vi "monitorRun.vi"(8 "error in (no error)":errorcluster) -> ()   [LabVIEW 2012]
uses:
  <vilib>/addons/database/Auxilliary.llb/DB Tools Cursor Type.ctl
  Global1.vi
  <vilib>/addons/database/Connection.llb/DB Tools Open Connec (Path).vi
  <vilib>/addons/database/Connection.llb/Conn Execute.vi
  <vilib>/addons/database/Recordset.llb/Rec Fetch Recordset Data (R).vi
  <vilib>/addons/database/Recordset.llb/Rec Destroy - Connection.vi
  <vilib>/addons/database/_DB Variant To Data/Database Variant To Data.xnode
  <vilib>/addons/database/NI_Database_API.lvlib
panel:
  out "error out":errorcluster
  out "M100 Monitor Board 2":string[][](table)
  in  "Table Control":string[][](table)
  out "error out 2":errorcluster
  in  "input cluster 2":T1
  in  "M100 Monitor Board":string[][](table)
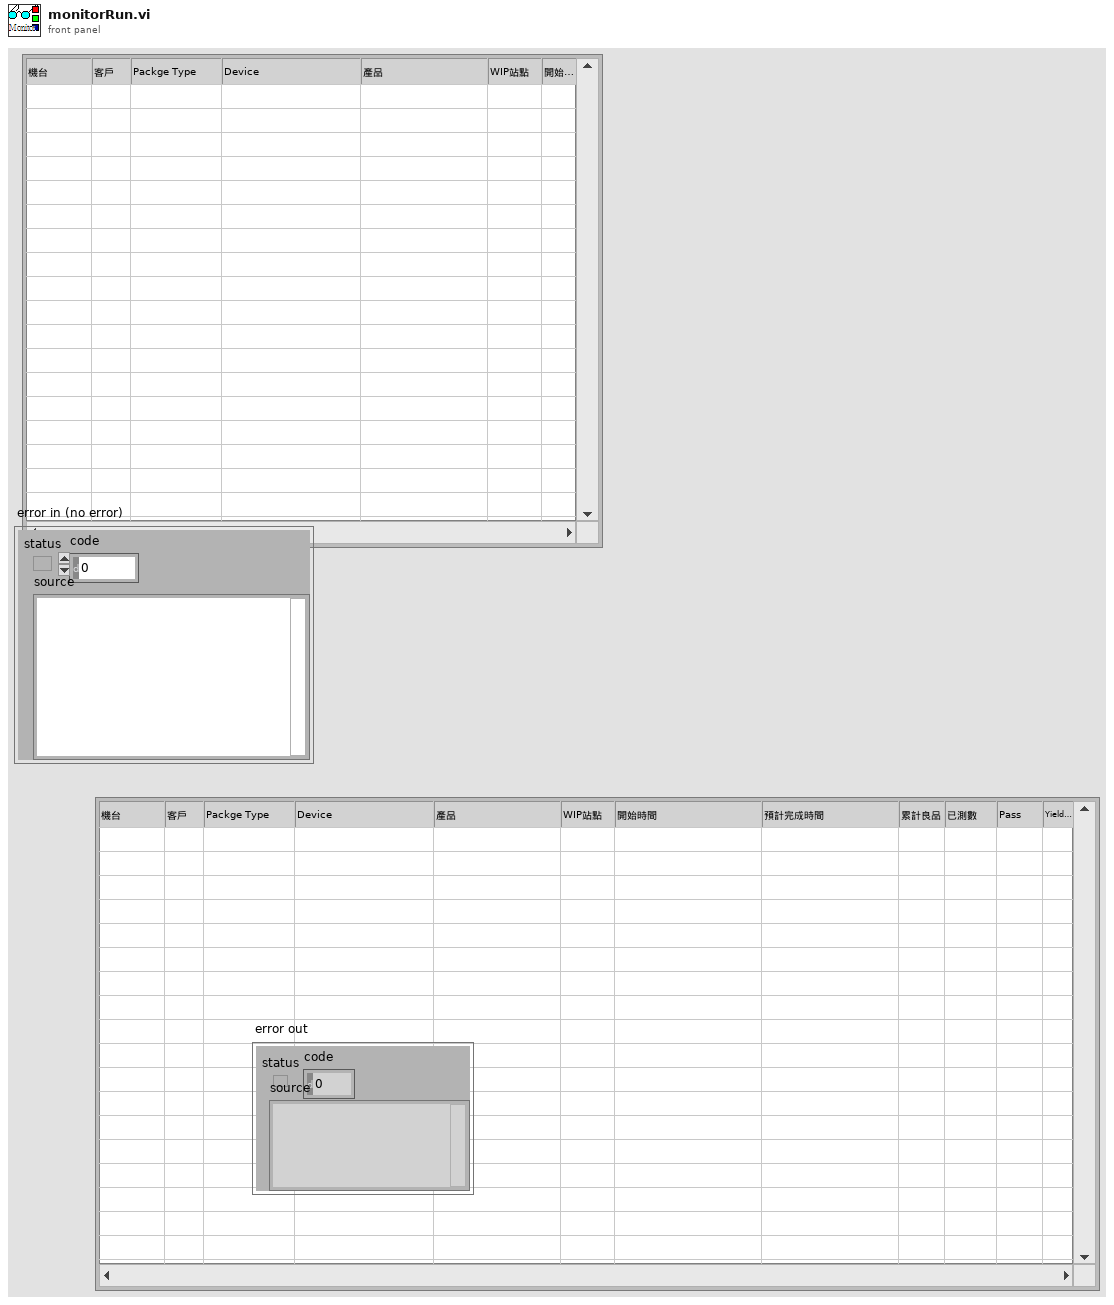
[diagram p1: front panel]
types:
  T1 = cluster{"Customer":string, "Package":string, "machine":string}
  T2 = typedef "NI_Database_API.lvlib/DB Tools Cursor Type.ctl" = enum16{"forward-only", "keyset", "dynamic", "static"}
  T3 = typedef "NI_Database_API.lvlib/Conn ObjectReference.ctl" = refnum<k1>
  T4 = typedef "LVDateTimeRec.ctl" = cluster{"fractional second":dbl, "second":i32, "minute":i32, "hour":i32, "day of month":i32, "month":i32, "year":i32, "day of week":i32, "day of year":i32, "DST":i32}
  T5 = typedef "LVRowAndColumnTypeDef.ctl" = cluster{"Row":i32, "Column":i32}
  T6 = typedef "NI_Database_API.lvlib/Rec ObjectReference.ctl" = refnum<k1>
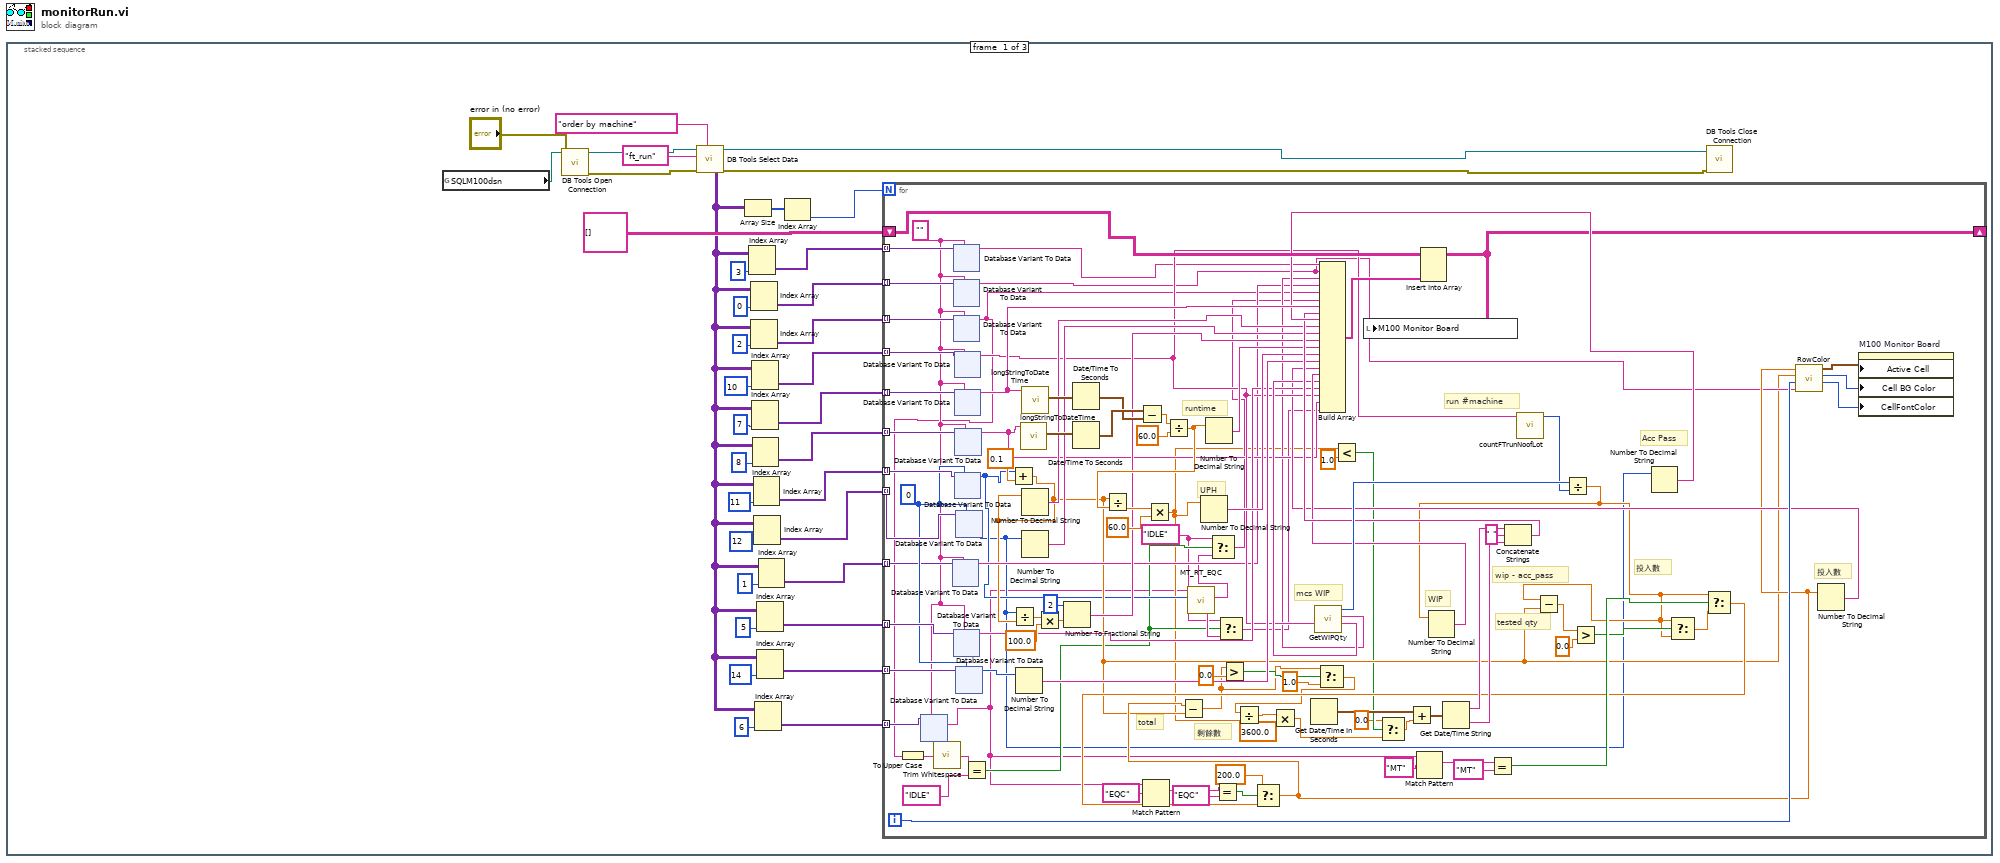
[diagram p0: block diagram]
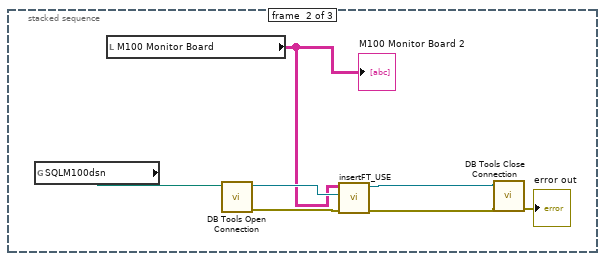
[diagram p2: hidden frame]
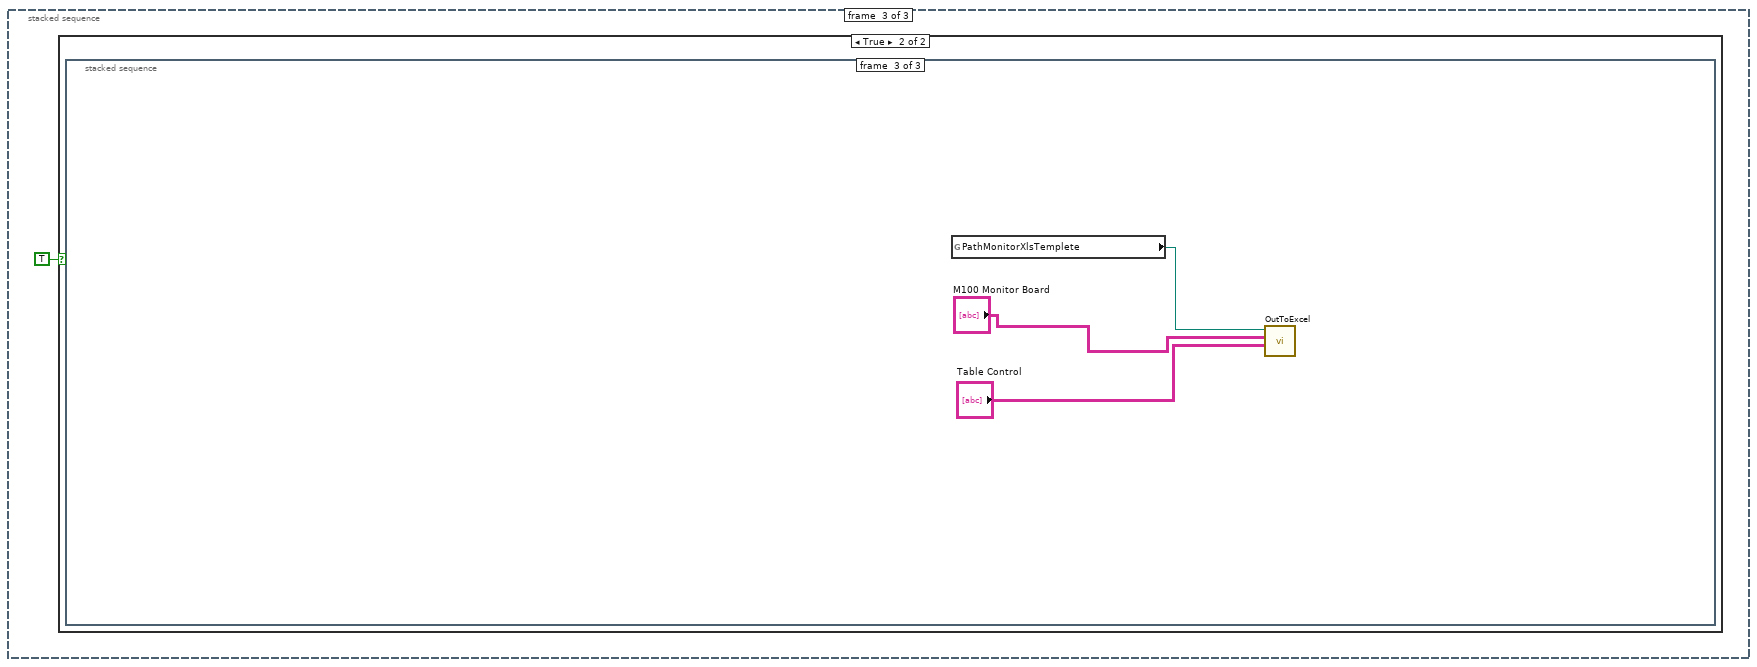
[diagram p3: hidden frame]
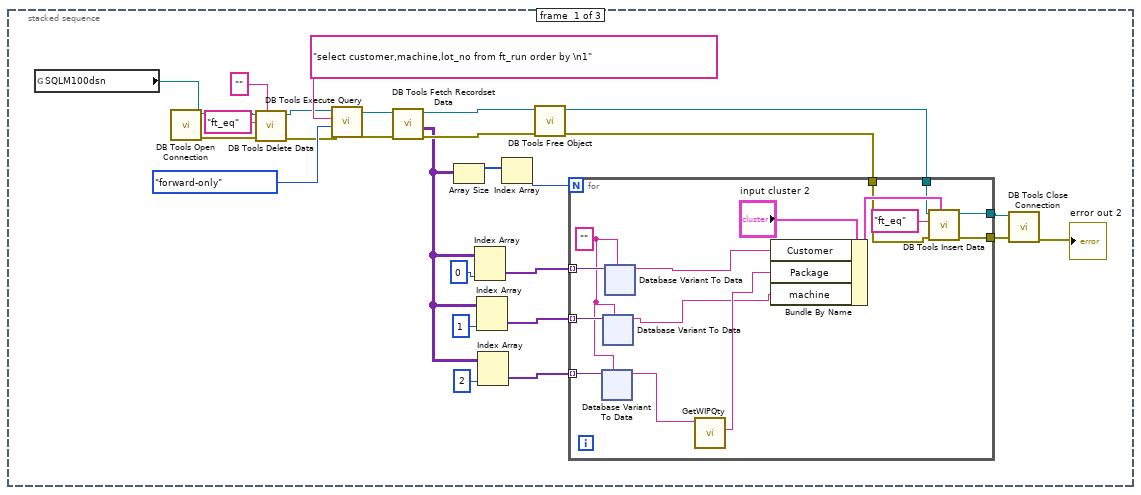
[diagram p5: hidden frame]
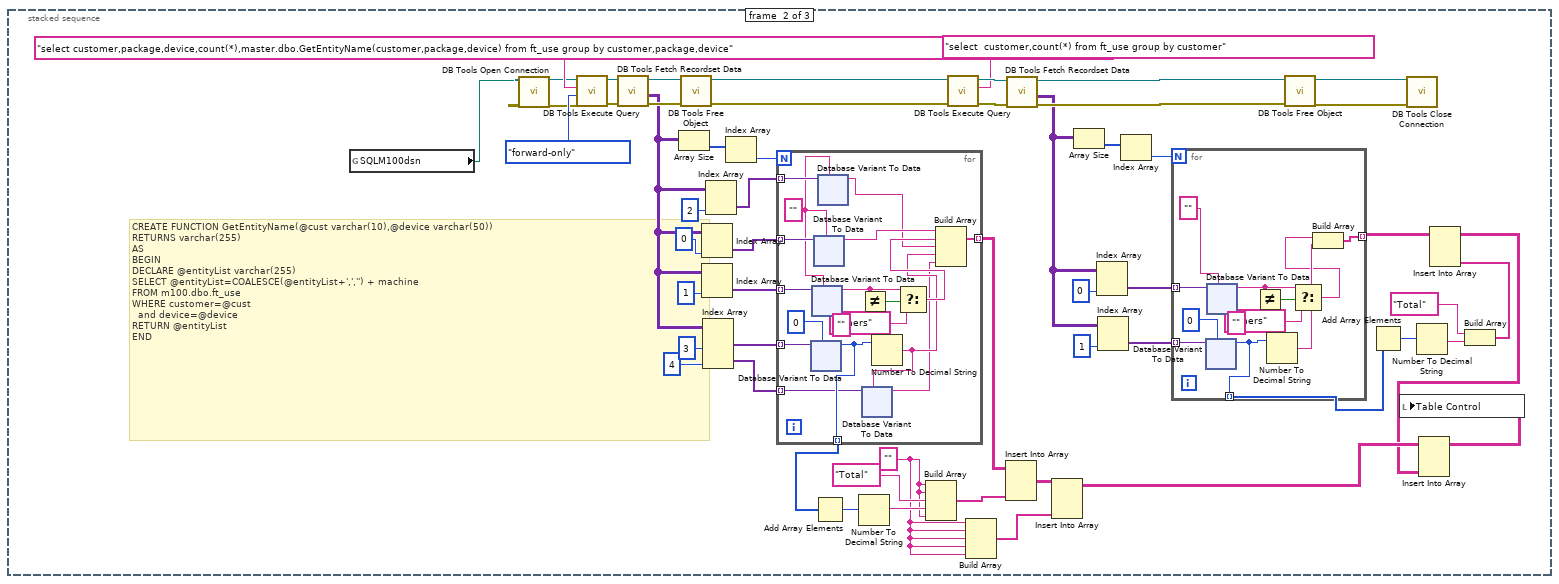
[diagram p6: hidden frame]
diagram:
  n1 = stacked-sequence {
    frame #0 {
      n2 = global read "Global1.vi" "SQLM100dsn"() -> (w4:path)
      n3 = call-poly <vilib>:"DB Tools Open Connection.vi"("error in (no error)"="error in (no error)", "connection information"=w4) -> ("error out"=w35:errorcluster, "connection reference"=w36:T3)  [unwired: 6 in]
      n4 = call <vilib>:"DB Tools Select Data.vi"("condition"="order by machine", "error in (no error)"=w35, "table"="ft_run", "connection reference"=w36) -> ("error out"=w6:errorcluster, "data"=w3:variant[][], "connection reference out"=w7:T3)  [unwired: 2 in]
      n5 = Array Size(array=w3) -> (size(s)=w33:i32[])
      n6 = Index Array(array=w3, index (col)=3) -> (element=w22:variant[])  [unwired: 1 in]
      n7 = Index Array(array=w3, index (col)=0) -> (element=w29:variant[])  [unwired: 1 in]
      n8 = Index Array(array=w3, index (col)=2) -> (element=w21:variant[])  [unwired: 1 in]
      n9 = Index Array(array=w3, index (col)=10) -> (element=w20:variant[])  [unwired: 1 in]
      n10 = Index Array(array=w3, index (col)=7) -> (element=w19:variant[])  [unwired: 1 in]
      n11 = Index Array(array=w3, index (col)=8) -> (element=w15:variant[])  [unwired: 1 in]
      n12 = Index Array(array=w3, index (col)=11) -> (element=w18:variant[])  [unwired: 1 in]
      n13 = Index Array(array=w3, index (col)=12) -> (element=w17:variant[])  [unwired: 1 in]
      n14 = Index Array(array=w3, index (col)=6 ("disabled index (col)")) -> (element=w1:variant[])  [unwired: 1 in]
      n15 = Index Array(array=w3, index (col)=5) -> (element=w13:variant[])  [unwired: 1 in]
      n16 = Index Array(array=w3, index (col)=14 ("disabled index (col)")) -> (element=w11:variant[])  [unwired: 1 in]
      n17 = Index Array(array=w3, index (col)=1 ("disabled index (col)")) -> (element=w8:variant[])  [unwired: 1 in]
      n18 = Index Array(array=w33) -> (element=w32:i32)  [unwired: 1 in]
      n19 = for {
        N: w32 -> [_]
        tunnel: w29 -> [w137] mode=indexing
        tunnel: w17 -> [w141] mode=indexing
        shift-right: [w72] -> _
        shift-left: string[][] [] -> [w140]
        tunnel: w22 -> [w138] mode=indexing
        tunnel: w21 -> [w136] mode=indexing
        tunnel: w20 -> [w135] mode=indexing
        tunnel: w19 -> [w134] mode=indexing
        tunnel: w18 -> [w133] mode=indexing
        tunnel: w15 -> [w129] mode=indexing
        tunnel: w13 -> [w119] mode=indexing
        tunnel: w11 -> [w118] mode=indexing
        tunnel: w8 -> [w77] mode=indexing
        tunnel: w1 -> [w58] mode=indexing
        i -> [w105]
        w50 = "IDLE" ("t")
        w117 = 0
        w57 = ""
        # "tested qty"
        # "wip - acc_pass"
        # "投入數"
        # "剩餘數"
        # "WIP"
        # "mcs WIP"
        # "run #machine"
        # "Acc Pass"
        # "total"
        # "UPH"
        # "runtime"
        # "投入數"
        n20 = xnode "Database Variant To Data"("database variant"=w58, "type"=w57) -> ("data"=w40:string)  [unwired: 1 in, 1 out]
        n21 = xnode "Database Variant To Data"("database variant"=w77, "type"=w57) -> ("data"=w73:string)  [unwired: 1 in, 1 out]
        n22 = xnode "Database Variant To Data"("database variant"=w138, "type"=w57) -> ("data"=w76:string)  [unwired: 1 in, 1 out]
        n23 = xnode "Database Variant To Data"("database variant"=w137, "type"=w57) -> ("data"=w75:string)  [unwired: 1 in, 1 out]
        n24 = xnode "Database Variant To Data"("database variant"=w136, "type"=w57) -> ("data"=w39:string)  [unwired: 1 in, 1 out]
        n25 = To Upper Case(1:w39) -> (0:w38:string)
        n26 = call <vilib>:"Trim Whitespace.vi"("string"=w38) -> ("trimmed string"=w37:string)  [unwired: 1 in]
        n27 = xnode "Database Variant To Data"("database variant"=w119, "type"=w57) -> ("data"=w91:string)  [unwired: 1 in, 1 out]
        n28 = xnode "Database Variant To Data"("database variant"=w135, "type"=w57) -> ("data"=w90:string)  [unwired: 1 in, 1 out]
        n29 = xnode "Database Variant To Data"("database variant"=w134, "type"=w57) -> ("data"=w102:string)  [unwired: 1 in, 1 out]
        n30 = xnode "Database Variant To Data"("database variant"=w133, "type"=w117) -> ("data"=w59:i32)  [unwired: 1 in, 1 out]
        n31 = xnode "Database Variant To Data"("database variant"=w129, "type"=w57) -> ("data"=w88:string)  [unwired: 1 in, 1 out]
        n32 = xnode "Database Variant To Data"("database variant"=w141, "type"=w117) -> ("data"=w45:i32)  [unwired: 1 in, 1 out]
        n33 = xnode "Database Variant To Data"("database variant"=w118, "type"=w117) -> ("data"=w116:i32)  [unwired: 1 in, 1 out]
        n34 = Equal?(x=w37, y="IDLE") -> (x = y?=w51:bool)
        n35 = Add(x=w59, y=0.1) -> (x+y=w65:dbl)
        n36 = Divide(x=w45, y=w65) -> (x/y=w130:dbl)
        n37 = Number To Decimal String(number=w116) -> (decimal integer string=w94:string)  [unwired: 1 in]
        n38 = call "longStringToDateTime.vi"("input string"=w88) -> ("output cluster"=w128:T4)  [unwired: 10 in]
        n39 = call "longStringToDateTime.vi"("input string"=w102) -> ("output cluster"=w127:T4)  [unwired: 10 in]
        n40 = Number To Decimal String(number=w65) -> (decimal integer string=w99:string)  [unwired: 1 in]
        n41 = Number To Decimal String(number=w45) -> (decimal integer string=w98:string)  [unwired: 1 in]
        n42 = Multiply(x=w130, y=100.0) -> (x*y=w131:dbl)
        n43 = Number To Fractional String(number=w131, precision (6)=i16 2) -> (F-format string=w97:string)  [unwired: 2 in]
        n44 = Date/Time To Seconds(2:w127) -> (0:w125:timestamp)  [unwired: 1 in]
        n45 = Date/Time To Seconds(2:w128) -> (0:w126:timestamp)  [unwired: 1 in]
        n46 = Subtract(x=w126, y=w125) -> (x-y=w124:dbl)
        n47 = Match Pattern(string=w40, regular expression="EQC") -> (match substring=w86:string)  [unwired: 1 in, 3 out]
        n48 = Divide(x=w124, y=60.0) -> (x/y=w122:dbl)
        n49 = Divide(x=w65, y=w122) -> (x/y=w121:dbl)
        n50 = Multiply(x=w121, y=60.0) -> (x*y=w48:dbl)
        n51 = call "MT_RT_EQC.vi"("Qty"=w59, "input string"=w40) -> ("Station"=w54:string, "STN"=w52:string)  [unwired: 5 in, 3 out]
        n52 = Number To Decimal String(number=w48) -> (decimal integer string=w95:string)  [unwired: 1 in]
        n53 = Number To Decimal String(number=w122) -> (decimal integer string=w96:string)  [unwired: 1 in]
        n54 = Select(t=w50, s=w51, f=w54) -> (s? t:f=w55:string)
        n55 = Equal?(x=w86, y="EQC") -> (x = y?=w84:bool)
        n56 = Select(t=w50, s=w51, f=w52) -> (s? t:f=w53:string)
        n57 = Get Date/Time In Seconds() -> (seconds since 1Jan1904=w113:timestamp)
        n58 = call "GetWIPQty.vi"("Lotno"=w90) -> ("lotno"=w92:string, "Package"=w74:string, "data"=w104:i32)  [unwired: 2 in, 6 out]
        n59 = Less?(x=w48, y=1.0) -> (x < y?=w44:bool)
        n60 = Match Pattern(string=w40, regular expression="MT") -> (match substring=w82:string)  [unwired: 1 in, 3 out]
        n61 = Equal?(x=w82, y="MT") -> (x = y?=w80:bool)
        n62 = call "countFTrunNoofLot.vi"("Lotno"=w90) -> ("data"=w103:i32)  [unwired: 10 in]
        n63 = Divide(x=w104, y=w103) -> (x/y=w49:dbl)
        n64 = Number To Decimal String(number=w49) -> (decimal integer string=w93:string)  [unwired: 1 in]
        n65 = Subtract(x=w49, y=w65) -> (x-y=w68:dbl)
        n66 = Greater?(x=w68, y=0.0) -> (0:w70:bool)
        n67 = Number To Decimal String(number=w45) -> (decimal integer string=w101:string)  [unwired: 1 in]
        n68 = Select(t=w49, s=w70, f=w49) -> (s? t:f=w69:dbl)
        n69 = Select(t=w49, s=w80, f=w69) -> (s? t:f=w79:dbl)
        n70 = Select(t=200.0, s=w84, f=w79) -> (s? t:f=w78:dbl)
        n71 = Subtract(x=w78, y=w65) -> (x-y=w62:dbl)
        n72 = Greater?(x=w62, y=0.0) -> (0:w63:bool)
        n73 = Select(t=w62, s=w63, f=1.0) -> (s? t:f=w60:dbl)
        n74 = Divide(x=w60, y=w48) -> (x/y=w115:dbl)
        n75 = Multiply(x=w115, y=3600.0) -> (x*y=w42:dbl)
        n76 = Select(t=0.0, s=w44, f=w42) -> (s? t:f=w41:dbl)
        n77 = Add(x=w113, y=w41) -> (x+y=w112:timestamp)
        n78 = Get Date/Time String(seconds (now)=w112) -> (date string=w111:string, time string=w110:string)  [unwired: 2 in]
        n79 = Concatenate Strings(w111, " " ("string"), w110) -> (w100:string)
        n80 = call "RowColor.vi"("Customer"=w75, "Row"=w105, "tested"=w65, "Input"=w78) -> ("FontColor"=w106:u32, "bgcolor"=w107:u32, "ActiveCell"=w108:T5)  [unwired: 5 in]
        n81 = Number To Decimal String(number=w78) -> (decimal integer string=w89:string)  [unwired: 1 in]
        n82 = Build Array(w76, w75, w74, w73, w39, w55, w102, w100, w101, w99, w98, w97, w96, w95, w94, w89, w93, w92, w91, w90, w88, w53) -> (w139:string[])
        n83 = Insert Into Array(array=w140, new element=w139) -> (w72:string[][])  [unwired: 2 in]
        n84 = local write "M100 Monitor Board"(w72) -> ()
        n85 = property on="M100 Monitor Board" class="Tbl (strict)"("Active Cell"=w108, "Cell BG Color"=w107, "CellFontColor"=w106) -> ()  [unwired: 2 in, 2 out]
      }
      n86 = call <vilib>:"DB Tools Close Connection.vi"("error in (no error)"=w6, "connection reference"=w7) -> ()  [unwired: 5 in, 1 out]
    }
    frame #1 {
      n87 = global read "Global1.vi" "SQLM100dsn"() -> (w529:path)
      n88 = local read "M100 Monitor Board"() -> (w528:string[][])
      "M100 Monitor Board 2" <- w528
      n89 = call-poly <vilib>:"DB Tools Open Connection.vi"("connection information"=w529) -> ("error out"=w531:errorcluster, "connection reference"=w532:T3)  [unwired: 7 in]
      n90 = call "insertFT_USE.vi"("M100 Monitor Board"=w528, "connection reference"=w532, "error in (no error)"=w531) -> ("connection reference out"=w530:T3, "error out"=w526:errorcluster)  [unwired: 6 in]
      n91 = call <vilib>:"DB Tools Close Connection.vi"("error in (no error)"=w526, "connection reference"=w530) -> ("error out"=→"error out":errorcluster)  [unwired: 5 in]
    }
    frame #2 {
      n92 = case shown="True" TRUE {
        frame False {
        }
        frame True {
          n93 = stacked-sequence {
            frame #0 {
              n94 = global read "Global1.vi" "SQLM100dsn"() -> (w534:path)
              n95 = call-poly <vilib>:"DB Tools Open Connection.vi"("connection information"=w534) -> ("error out"=w545:errorcluster, "connection reference"=w546:T3)  [unwired: 7 in]
              n96 = call <vilib>:"DB Tools Delete Data.vi"("condition"="", "error in (no error)"=w545, "table"="ft_eq", "connection reference"=w546) -> ("error out"=w543:errorcluster, "connection reference out"=w542:T3)  [unwired: 6 in]
              n97 = call-poly <vilib>:"DB Tools Execute Query.vi"("error in (no error)"=w543, "cursor type"=DB_Tools_Cursor_Type."forward-only", "SQL query"="select customer,machine,lot_no from ft_run order by \n1", "connection reference"=w542) -> ("error out"=w558:errorcluster, "recordset reference"=w560:T6)  [unwired: 4 in]
              n98 = call-poly <vilib>:"DB Tools Fetch Recordset Data.vi"("error in (no error)"=w558, "recordset reference"=w560) -> ("error out"=w557:errorcluster, "recordset data"=w552:variant[][], "recordset reference out"=w559:T6)  [unwired: 3 in]
              n99 = Array Size(array=w552) -> (size(s)=w551:i32[])
              n100 = Index Array(array=w552, index (col)=0 ("disabled index (col)")) -> (element=w549:variant[])  [unwired: 1 in]
              n101 = Index Array(array=w552, index (col)=1 ("disabled index (col)")) -> (element=w548:variant[])  [unwired: 1 in]
              n102 = Index Array(array=w552, index (col)=2) -> (element=w547:variant[])  [unwired: 1 in]
              n103 = Index Array(array=w551) -> (element=w550:i32)  [unwired: 1 in]
              n104 = call-poly <vilib>:"DB Tools Free Object.vi"("error in (no error)"=w557, "recordset reference"=w559) -> ("error out"=w538:errorcluster, "connection reference"=w539:T3)  [unwired: 8 in]
              n105 = for {
                N: w550 -> [_]
                tunnel: w549 -> [w575] mode=indexing
                tunnel: w548 -> [w574] mode=indexing
                tunnel: w547 -> [w573] mode=indexing
                tunnel: w539 -> [w564]
                tunnel: w538 -> [w563]
                tunnel: [w562] -> w537
                tunnel: [w561] -> w536
                w572 = ""
                n106 = xnode "Database Variant To Data"("database variant"=w573, "type"=w572) -> ("data"=w571:string)  [unwired: 1 in, 1 out]
                n107 = xnode "Database Variant To Data"("database variant"=w574, "type"=w572) -> ("data"=w566:string)  [unwired: 1 in, 1 out]
                n108 = xnode "Database Variant To Data"("database variant"=w575, "type"=w572) -> ("data"=w568:string)  [unwired: 1 in, 1 out]
                n109 = call "GetWIPQty.vi"("Lotno"=w571) -> ("Package"=w567:string)  [unwired: 2 in, 8 out]
                n110 = Bundle By Name(cluster="input cluster 2", "Customer"=w568, "Package"=w567, "machine"=w566) -> (w565:T1)
                n111 = call <vilib>:"DB Tools Insert Data.vi"("data"=w565, "error in (no error)"=w563, "table"="ft_eq", "connection reference"=w564) -> ("error out"=w561:errorcluster, "connection reference out"=w562:T3)  [unwired: 6 in]
              }
              n112 = call <vilib>:"DB Tools Close Connection.vi"("error in (no error)"=w536, "connection reference"=w537) -> ("error out"=→"error out 2":errorcluster)  [unwired: 5 in]
            }
            frame #1 {
              w672 = "" ("element")
              # "CREATE FUNCTION GetEntityName(@cust varchar(10),@device varchar(50))\nRETURNS varchar(255) \nAS\nBEGIN\nDECLARE @entityList varchar(255)\nSELECT @entityList=COALESCE(@entityList+',','') + machine\nFROM m100.dbo.ft_use\nWHERE customer=@cust\n  and device=@device\nRETURN @entityList\nEND"
              n113 = global read "Global1.vi" "SQLM100dsn"() -> (w675:path)
              n114 = call-poly <vilib>:"DB Tools Open Connection.vi"("connection information"=w675) -> ("error out"=w716:errorcluster, "connection reference"=w717:T3)  [unwired: 7 in]
              n115 = call-poly <vilib>:"DB Tools Execute Query.vi"("error in (no error)"=w716, "cursor type"=DB_Tools_Cursor_Type."forward-only", "SQL query"="select customer,package,device,count(*),master.dbo.GetEntityName(customer,package,device) from ft_use group by customer,package,device", "connection reference"=w717) -> ("error out"=w725:errorcluster, "recordset reference"=w727:T6)  [unwired: 4 in]
              n116 = call-poly <vilib>:"DB Tools Fetch Recordset Data.vi"("error in (no error)"=w725, "recordset reference"=w727) -> ("error out"=w724:errorcluster, "recordset data"=w678:variant[][], "recordset reference out"=w726:T6)  [unwired: 3 in]
              n117 = Array Size(array=w678) -> (size(s)=w719:i32[])
              n118 = call-poly <vilib>:"DB Tools Free Object.vi"("error in (no error)"=w724, "recordset reference"=w726) -> ("error out"=w685:errorcluster, "connection reference"=w686:T3)  [unwired: 8 in]
              n119 = Index Array(array=w678, index (col)=0 ("disabled index (col)")) -> (element=w714:variant[])  [unwired: 1 in]
              n120 = Index Array(array=w678, index (col)=1 ("disabled index (col)")) -> (element=w713:variant[])  [unwired: 1 in]
              n121 = Index Array(array=w678, index (col) #1=3 ("index (col)"), index (col) #2=4 ("index (col)")) -> (element #1=w712:variant[], element #2=w673:variant[])  [unwired: 2 in]
              n122 = Index Array(array=w678, index (col)=2 ("disabled index (col)")) -> (element=w676:variant[])  [unwired: 1 in]
              n123 = Index Array(array=w719) -> (element=w715:i32)  [unwired: 1 in]
              n124 = for {
                N: w715 -> [_]
                tunnel: w714 -> [w821] mode=indexing
                tunnel: w713 -> [w820] mode=indexing
                tunnel: w712 -> [w819] mode=indexing
                tunnel: [w816] -> w707 mode=indexing
                tunnel: [w810] -> w710 mode=indexing
                tunnel: w676 -> [w809] mode=indexing
                tunnel: w673 -> [w806] mode=indexing
                w808 = ""
                n125 = xnode "Database Variant To Data"("database variant"=w819, "type"=0) -> ("data"=w810:i32)  [unwired: 1 in, 1 out]
                n126 = xnode "Database Variant To Data"("database variant"=w820, "type"=w808) -> ("data"=w813:string)  [unwired: 1 in, 1 out]
                n127 = xnode "Database Variant To Data"("database variant"=w821, "type"=w808) -> ("data"=w817:string)  [unwired: 1 in, 1 out]
                n128 = xnode "Database Variant To Data"("database variant"=w809, "type"=w808) -> ("data"=w807:string)  [unwired: 1 in, 1 out]
                n129 = Not Equal?(x=w813, y="") -> (x != y?=w814:bool)
                n130 = Number To Decimal String(number=w810) -> (decimal integer string=w805:string)  [unwired: 1 in]
                n131 = xnode "Database Variant To Data"("database variant"=w806, "type"=w805) -> ("data"=w804:string)  [unwired: 1 in, 1 out]
                n132 = Select(t=w813, s=w814, f="Others") -> (s? t:f=w811:string)
                n133 = Build Array(w817, w811, w807, w805, w804) -> (w816:string[])
              }
              n134 = Add Array Elements(numeric array=w710) -> (sum=w711:i32)
              n135 = Number To Decimal String(number=w711) -> (decimal integer string=w709:string)  [unwired: 1 in]
              n136 = Build Array(w672, w672, "Total" ("element"), w709, w672) -> (w706:string[])
              n137 = call-poly <vilib>:"DB Tools Execute Query.vi"("error in (no error)"=w685, "SQL query"="select  customer,count(*) from ft_use group by customer", "connection reference"=w686) -> ("error out"=w703:errorcluster, "recordset reference"=w705:T6)  [unwired: 5 in]
              n138 = Build Array(w672, w672, w672, w672, w672) -> (w687:string[])
              n139 = Insert Into Array(array=w707, new element=w706) -> (w688:string[][])  [unwired: 2 in]
              n140 = call-poly <vilib>:"DB Tools Fetch Recordset Data.vi"("error in (no error)"=w703, "recordset reference"=w705) -> ("error out"=w702:errorcluster, "recordset data"=w699:variant[][], "recordset reference out"=w704:T6)  [unwired: 3 in]
              n141 = Insert Into Array(array=w688, new element=w687) -> (w681:string[][])  [unwired: 2 in]
              n142 = Array Size(array=w699) -> (size(s)=w698:i32[])
              n143 = Index Array(array=w699, index (col)=0 ("disabled index (col)")) -> (element=w696:variant[])  [unwired: 1 in]
              n144 = Index Array(array=w699, index (col)=1) -> (element=w695:variant[])  [unwired: 1 in]
              n145 = Index Array(array=w698) -> (element=w697:i32)  [unwired: 1 in]
              n146 = for {
                N: w697 -> [_]
                tunnel: w696 -> [w738] mode=indexing
                tunnel: w695 -> [w737] mode=indexing
                tunnel: [w734] -> w690 mode=indexing
                tunnel: [w728] -> w693 mode=indexing
                n147 = xnode "Database Variant To Data"("database variant"=w737, "type"=0) -> ("data"=w728:i32)  [unwired: 1 in, 1 out]
                n148 = xnode "Database Variant To Data"("database variant"=w738, "type"="") -> ("data"=w731:string)  [unwired: 1 in, 1 out]
                n149 = Not Equal?(x=w731, y="") -> (x != y?=w732:bool)
                n150 = Number To Decimal String(number=w728) -> (decimal integer string=w735:string)  [unwired: 1 in]
                n151 = Select(t=w731, s=w732, f="Others") -> (s? t:f=w729:string)
                n152 = Build Array(w729, w735) -> (w734:string[])
              }
              n153 = call-poly <vilib>:"DB Tools Free Object.vi"("error in (no error)"=w702, "recordset reference"=w704) -> ("error out"=w683:errorcluster, "connection reference"=w684:T3)  [unwired: 8 in]
              n154 = Add Array Elements(numeric array=w693) -> (sum=w694:i32)
              n155 = call <vilib>:"DB Tools Close Connection.vi"("error in (no error)"=w683, "connection reference"=w684) -> ()  [unwired: 5 in, 1 out]
              n156 = Number To Decimal String(number=w694) -> (decimal integer string=w692:string)  [unwired: 1 in]
              n157 = Build Array("Total" ("element"), w692) -> (w689:string[])
              n158 = Insert Into Array(array=w690, new element=w689) -> (w680:string[][])  [unwired: 2 in]
              n159 = Insert Into Array(array=w681, new element=w680) -> (w679:string[][])  [unwired: 2 in]
              n160 = local write "Table Control"(w679) -> ()
            }
            frame #2 {
              n161 = global read "Global1.vi" "PathMonitorXlsTemplete"() -> (w982:path)
              n162 = call "OutToExcel.vi"("Table Control"="Table Control", "Running"="M100 Monitor Board", "Report Template"=w982) -> ()  [unwired: 9 in]
            }
          }
        }
      }
    }
  }
